vi "Write UID.vi"(8 "error in (no error)":errorcluster, 10 "UID":string, 11 "Document in":refnum<class "Document.lvclass">) -> (0 "error out":errorcluster, 3 "Document out":refnum<class "Document.lvclass">)   [LabVIEW 2016, in "Document.lvclass"]
uses:
  Document.lvclass
  Document.lvclass/Document.ctl
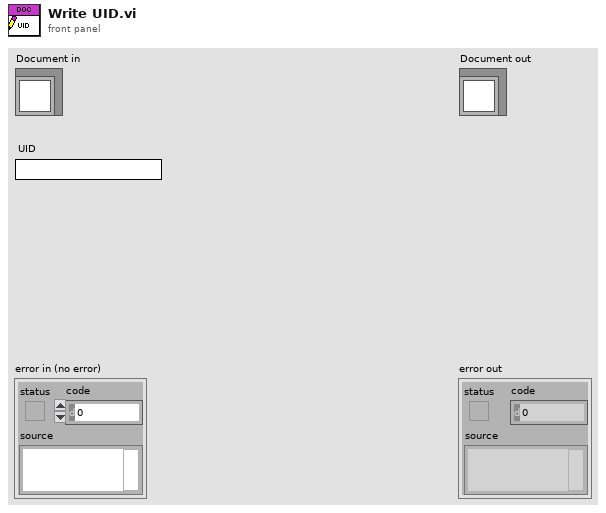
[diagram p1: front panel]
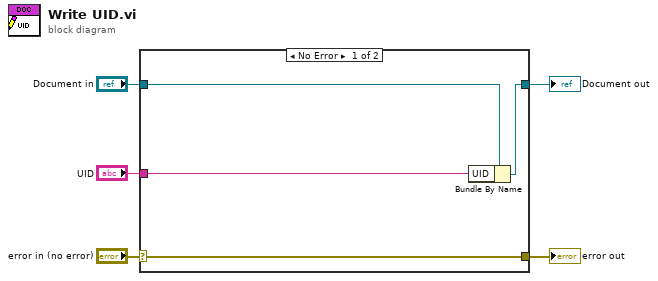
[diagram p0: block diagram]
diagram:
  n1 = case shown="No Error" "error in (no error)" {
    selector: "error in (no error)" -> [w9 w10]
    tunnel: [w9 w10] -> w4
    tunnel: [w7 w11] -> w2
    tunnel: "Document in" -> [w8 w11]
    tunnel: "UID" -> [w6 _]
    frame No Error {
      n2 = Bundle By Name(cluster=w8, "UID"=w6) -> (w7:refnum<class "Document.lvclass">)
    }
    frame Error {
    }
  }
  "error out" <- w4
  "Document out" <- w2
